vi "Create.vi"(8 "error in (no error)":errorcluster) -> (0 "error out":errorcluster, 3 "CT-De-energizeThenStop-Cmd out":refnum<class "CT-De-energizeThenStop-Cmd.lvclass">)   [LabVIEW 2013, in "CT-De-energizeThenStop-Cmd.lvclass"]
uses:
  CT-De-energizeThenStop-Cmd.lvclass
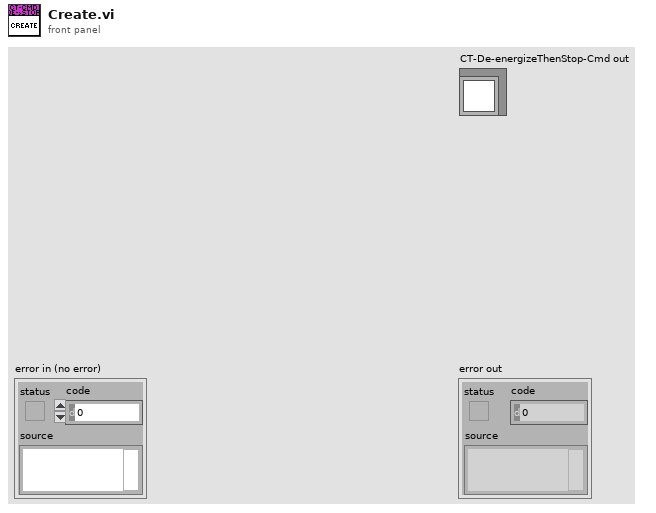
[diagram p1: front panel]
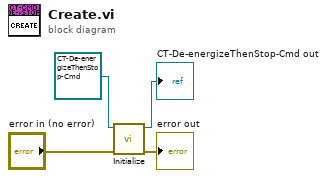
[diagram p0: block diagram]
diagram:
  n1 = call-dynamic "Initialize.vi"("error in (no error)"="error in (no error)", "CT-De-energizeThenStop-Cmd in"=refnum<class "CT-De-energizeThenStop-Cmd.lvclass"> refnum ("CT-De-energizeThenStop-Cmd.lvclass")) -> ("error out"=→"error out":errorcluster, "CT-De-energizeThenStop-Cmd out"=→"CT-De-energizeThenStop-Cmd out":refnum<class "CT-De-energizeThenStop-Cmd.lvclass">)  [unwired: 8 in]
